vi "Keithley 3390 Software Triggered Frequency Sweep.vi"() -> ()   [LabVIEW 2017]
doc: "This example shows how to configure and enable a triggered frequency sweep."
uses:
  Keithley 3390.lvlib
  Public/Configure/Configure Waveform (Sine).vi
panel:
  in  "Stop  Frequency  (1000.0 Hz)":dbl=1000.0 format="%#.6g"
  in  "Start Frequency (100.0 Hz)":dbl=100.0 format="%#.6g"
  in  "Sweep Time (1.00 s)":dbl=1.0 format="%#.6g"
  in  "Amplitude (1.0 Vpp)":dbl=1.0
  in  "VISA resource name":refnum<visa-resource-name>
  # "(c) 2008 Keithley Instruments, Inc.  ALL RIGHTS RESERVED."
  # "In this example the function generator\nis configured to output a sine wave\nand perform a frequency sweep.  The\ntrigger mode is set to Bus (Software).\n\nThe example then sends out triggers\nonce every 3 seconds, five times.\nNotice how the Sweep Time long\nsweeps start every 3 seconds."
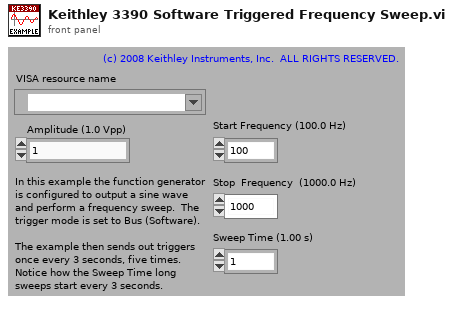
[diagram p1: front panel]
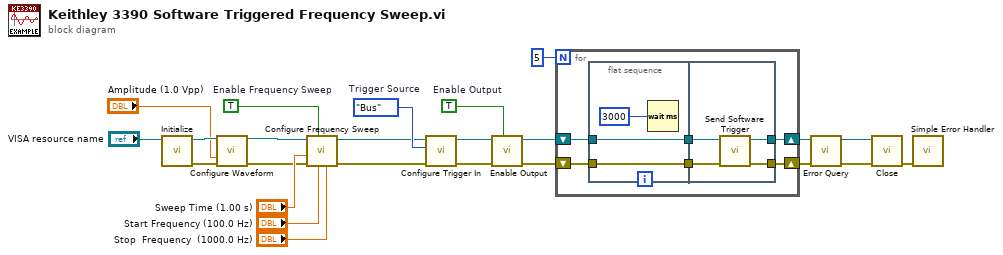
[diagram p0: block diagram]
diagram:
  w7 = enum16{"Immediate", "External", "Bus"}."Bus"  # Trigger Source
  w8 = TRUE  # Enable Output
  w20 = TRUE  # Enable Frequency Sweep
  n1 = call "Initialize.vi"("VISA resource name"="VISA resource name") -> ("error out"=w21:errorcluster, "VISA resource name out"=w24:refnum<visa-resource-name>)  [unwired: 9 in]
  n2 = call-poly "Configure Waveform.vi"("VISA resource name"=w24, "Amplitude (1.0 Vpp)"="Amplitude (1.0 Vpp)", "error in (no error)"=w21) -> ("VISA resource name out"=w2:refnum<visa-resource-name>, "error out"=w1:errorcluster)  [unwired: 11 in]
  n3 = call "Configure Frequency Sweep.vi"("Stop  Frequency  (1000.0 Hz)"="Stop  Frequency  (1000.0 Hz)", "Start Frequency (100.0 Hz)"="Start Frequency (100.0 Hz)", "Enable Frequency Sweep (T:Enable)"=w20, "error in (no error)"=w1, "Sweep Time (1.00 s)"="Sweep Time (1.00 s)", "VISA resource name"=w2) -> ("error out"=w6:errorcluster, "VISA resource name out"=w5:refnum<visa-resource-name>)  [unwired: 4 in]
  n4 = call "Configure Trigger In.vi"("error in (no error)"=w6, "Trigger Source (0:Immediate)"=w7, "VISA resource name"=w5) -> ("error out"=w3:errorcluster, "VISA resource name out"=w4:refnum<visa-resource-name>)  [unwired: 7 in]
  n5 = call "Enable Output.vi"("Enable Output (T: Enable)"=w8, "error in (no error)"=w3, "VISA resource name"=w4) -> ("error out"=w13:errorcluster, "VISA resource name out"=w19:refnum<visa-resource-name>)  [unwired: 7 in]
  n6 = for {
    N: 5 -> [_]
    shift-right: [w28] -> w10
    shift-left: w13 -> [w27]
    shift-right: [w29] -> w12
    shift-left: w19 -> [w30]
    n7 = flat-sequence {
      tunnel: w27 -> [w32]
      tunnel: w30 -> [w33]
      tunnel: [w33] -> w26
      tunnel: [w32] -> w25
      tunnel: [w36] -> w29
      tunnel: [w35] -> w28
      tunnel: w26 -> [w37]
      tunnel: w25 -> [w34]
      frame #0 {
        n8 = Wait (ms)(milliseconds to wait=u32 3000 ("millisecond multiple")) -> ()  [unwired: 1 out]
      }
      frame #1 {
        n9 = call "Send Software Trigger.vi"("error in (no error)"=w34, "VISA resource name"=w37) -> ("error out"=w35:errorcluster, "VISA resource name out"=w36:refnum<visa-resource-name>)  [unwired: 8 in]
      }
    }
  }
  n10 = call "Error Query.vi"("error in (no error)"=w10, "VISA resource name"=w12) -> ("error out"=w9:errorcluster, "VISA resource name out"=w11:refnum<visa-resource-name>)  [unwired: 6 in, 2 out]
  n11 = call "Close.vi"("error in (no error)"=w9, "VISA resource name"=w11) -> ("error out"=w23:errorcluster)  [unwired: 9 in]
  n12 = call <vilib>:"Simple Error Handler.vi"("error in (no error)"=w23) -> ()  [unwired: 4 in, 5 out]
